vi "Main.vi"() -> ()   [LabVIEW 2014]
uses:
  Person Data.ctl
  <vilib>/Utility/config.llb/Read Key (String).vi
  <vilib>/Utility/config.llb/NI_LVConfig.lvlib
panel:
  out "file path":path
  out "error out":errorcluster
  in  "NumberOfPerson":u32
  out "PersonData":T1={"Age"=18, "Name"="Noname", "Gender"=enum."Female"}
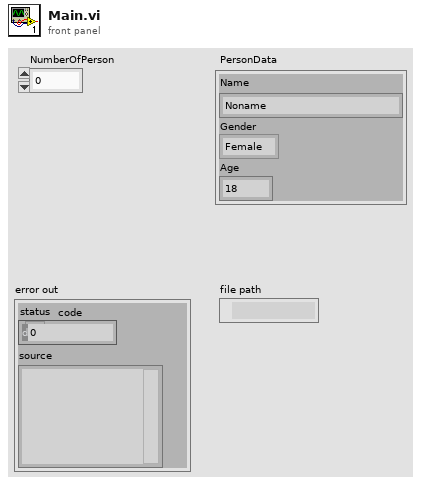
[diagram p1: front panel]
types:
  T1 = typedef "Person Data.ctl" = cluster{"Age":u32, "Name":string, "Gender":enum16{"Female", "Male", ""}}
  T2 = typedef "NI_LVConfig.lvlib/Config Data RefNum.ctl" = refnum<k1>
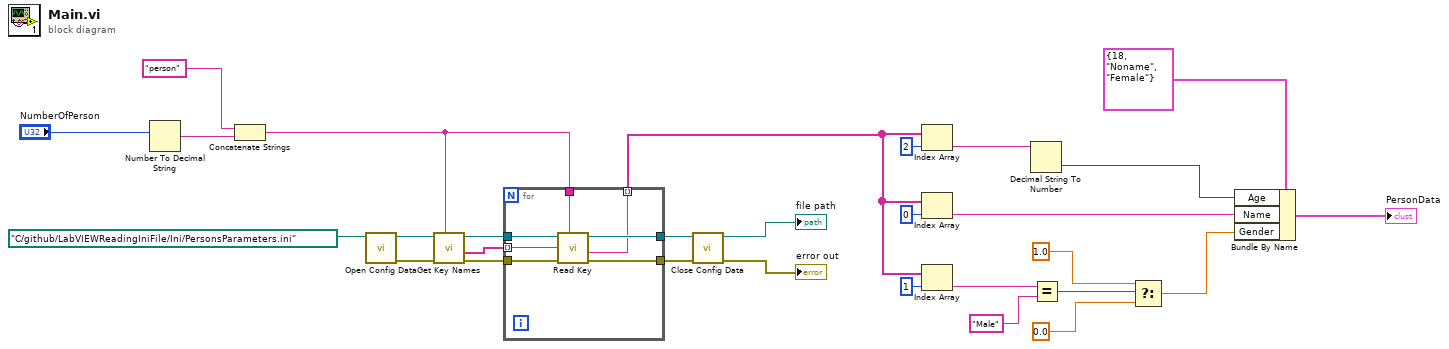
[diagram p0: block diagram]
diagram:
  n1 = Number To Decimal String(number="NumberOfPerson") -> (decimal integer string=w28:string)  [unwired: 1 in]
  n2 = Concatenate Strings("person", w28) -> (w20:string)
  n3 = call <vilib>:"Open Config Data.vi"("configuration file path"=path "C:/github/LabVIEWReadingIniFile/Ini/PersonsParameters.ini") -> ("error out"=w22:errorcluster, "refnum"=w23:T2)  [unwired: 8 in, 1 out]
  n4 = call <vilib>:"Get Key Names.vi"("section"=w20, "error in (no error)"=w22, "refnum"=w23) -> ("error out"=w21:errorcluster, "key names"=w18:string[], "refnum out"=w19:T2)  [unwired: 5 in, 1 out]
  n5 = for {
    tunnel: w21 -> [w36]
    tunnel: w20 -> [w35]
    tunnel: w19 -> [w34]
    tunnel: w18 -> [w33] mode=indexing
    tunnel: [w32] -> w16
    tunnel: [w31] -> w15
    tunnel: [w30] -> w14 mode=indexing
    n6 = call-poly <vilib>:"Read Key.vi"("section"=w35, "error in (no error)"=w36, "key"=w33, "refnum"=w34) -> ("error out"=w31:errorcluster, "value"=w30:string, "refnum out"=w32:T2)  [unwired: 4 in, 1 out]
  }
  n7 = call <vilib>:"Close Config Data.vi"("error in (no error)"=w15, "refnum"=w16) -> ("error out"=→"error out":errorcluster, "file path"=→"file path":path)  [unwired: 8 in]
  n8 = Index Array(array=w14, index=2) -> (element=w10:string)
  n9 = Index Array(array=w14, index=0) -> (element=w9:string)
  n10 = Index Array(array=w14, index=1) -> (element=w8:string)
  n11 = Decimal String To Number(string=w10) -> (number=w1:i32)  [unwired: 2 in, 1 out]
  n12 = Equal?(x=w8, y="Male") -> (x = y?=w6:bool)
  n13 = Select(t=1.0, s=w6, f=0.0) -> (s? t:f=w3:dbl)
  n14 = Bundle By Name(cluster=T1 {"Age"=18, "Name"="Noname", "Gender"=enum."Female"} ("PersonData"), "Age"=w1, "Name"=w9, "Gender"=w3) -> (→"PersonData":T1)
